vi "UpdateCommunicationStatus.vi"(1 "Block Diagram Control Enum":T1, 2 "Communication Enum Refnum in":refnum<vi>) -> ()   [LabVIEW 2015]
uses:
  CommunicationStatus.ctl
  BlockDiagramControlEnum.ctl
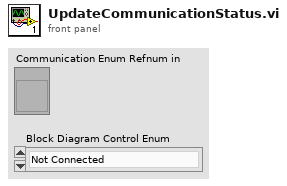
[diagram p1: front panel]
types:
  T1 = typedef "BlockDiagramControlEnum.ctl" = enum16{"Not Connected", "Disconnected", "Functional Test A", "Functional Test B", "Functional Test C", "Functional Test D", "Flight"}
  T2 = typedef "CommunicationStatus.ctl" = enum16{"Connected", "Disconnected"}
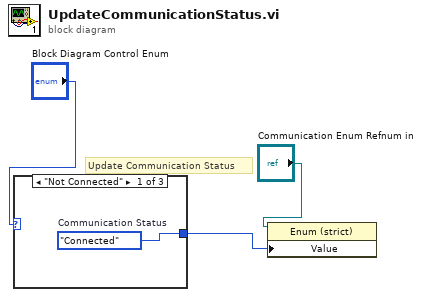
[diagram p0: block diagram]
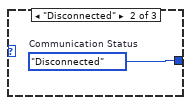
[diagram p2: hidden frame]
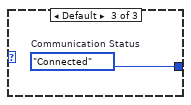
[diagram p3: hidden frame]
diagram:
  # "Update Communication Status"
  n1 = case shown="\"Not Connected\"" "Block Diagram Control Enum" {
    tunnel: [w4 w5 w6] -> w2
    frame "Not Connected" {
      w4 = CommunicationStatus."Connected"  # Communication Status
    }
    frame "Disconnected" {
      w5 = CommunicationStatus."Disconnected"  # Communication Status
    }
    frame Default {
      w6 = CommunicationStatus."Connected"  # Communication Status
    }
  }
  n2 = property class="Enum (strict)"(reference="Communication Enum Refnum in", "Value"=w2) -> ()  [unwired: 1 in, 2 out]
